vi "State.vi"(7 "Set (f)":bool, 11 "State":string) -> (3 "State":string)   [LabVIEW 2014, in "SyncModule.lvlib"]
uses:
  SyncModule.lvlib
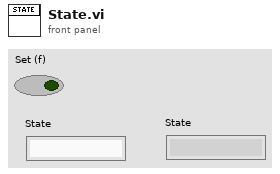
[diagram p1: front panel]
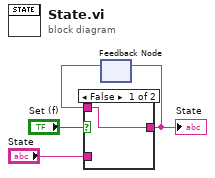
[diagram p0: block diagram]
diagram:
  n1 = feedback #1() -> (w1:string)  [unwired: 1 in]
  n2 = case shown="False" "Set (f)" {
    tunnel: "State" -> [_ w6]
    tunnel: [w5 w6] -> w2
    tunnel: w1 -> [w5 _]
    frame False {
    }
    frame True {
    }
  }
  "State" <- w2
  n3 = feedback-in #1(w2) -> ()
